vi "Comprobaciones.vi"() -> ()   [LabVIEW 2022 SP3]
panel:
  out "N^3=(N+1)/(N-1)":bool
  out "N-1=1/N":bool
  # "Comprobaciones"
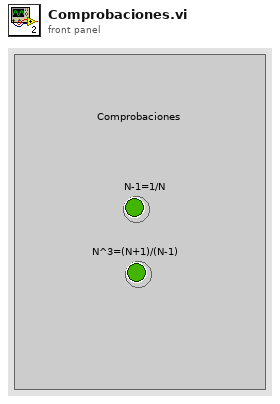
[diagram p1: front panel]
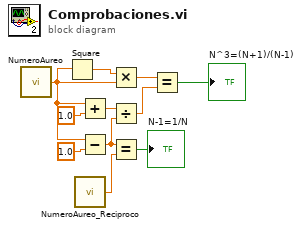
[diagram p0: block diagram]
diagram:
  n1 = call "NumeroAureo.vi"() -> ("Numero aureo"=w7:dbl)
  n2 = Square(x=w7) -> (x^2=w8:dbl)
  n3 = call "NumeroAureo_Reciproco.vi"() -> ("Recíproco"=w10:dbl)
  n4 = Add(x=w7, y=1.0) -> (x+y=w5:dbl)
  n5 = Subtract(x=w7, y=1.0) -> (x-y=w4:dbl)
  n6 = Multiply(x=w8, y=w7) -> (x*y=w3:dbl)
  n7 = Divide(x=w5, y=w4) -> (x/y=w2:dbl)
  n8 = Equal?(x=w4, y=w10) -> (x = y?=→"N-1=1/N":bool)
  n9 = Equal?(x=w3, y=w2) -> (x = y?=→"N^3=(N+1)/(N-1)":bool)
